vi "newTargetPos(Step).vi"(11 "Tapedrive_ESP301 in":refnum<class "Tapedrive_ESP301.lvclass">) -> (2 "String":string, 3 "Tapedrive_ESP301 out":refnum<class "Tapedrive_ESP301.lvclass">)   [LabVIEW 2013, in "Tapedrive_ESP301.lvclass"]
uses:
  Tapedrive_ESP301.lvclass
  Tapedrive_ESP301.lvclass/Tapedrive_ESP301.ctl
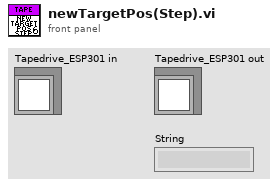
[diagram p1: front panel]
types:
  T1 = typedef "Direction.ctl" = enum16{"Forward", "Backward", "Undefined"}
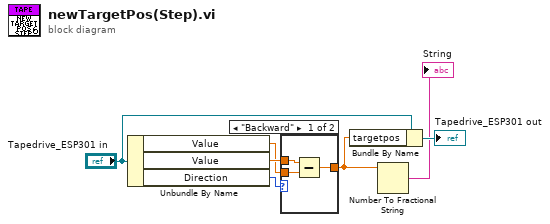
[diagram p0: block diagram]
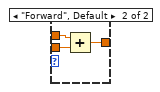
[diagram p2: hidden frame]
diagram:
  n1 = Unbundle By Name("Tapedrive_ESP301 in") -> ("Value"=w4:dbl, "Value"=w5:dbl, "Direction"=w3:T1)
  n2 = case shown="\"Backward\"" w3 {
    tunnel: w5 -> [w10 w12]
    tunnel: w4 -> [w9 w13]
    tunnel: [w8 w11] -> w2
    frame "Backward" {
      n3 = Subtract(x=w10, y=w9) -> (x-y=w8:dbl)
    }
    frame "Forward", Default {
      n4 = Add(x=w12, y=w13) -> (x+y=w11:dbl)
    }
  }
  n5 = Bundle By Name(cluster="Tapedrive_ESP301 in", "targetpos"=w2) -> (→"Tapedrive_ESP301 out":refnum<class "Tapedrive_ESP301.lvclass">)
  n6 = Number To Fractional String(number=w2) -> (F-format string=→"String":string)  [unwired: 3 in]
